vi "SubVI Nivel a Caudal peristaltica.vi"(11 "UInt16":u16) -> (3 "Numeric":dbl)   [LabVIEW 2013]
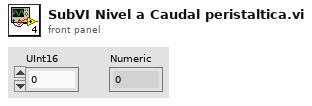
[diagram p1: front panel]
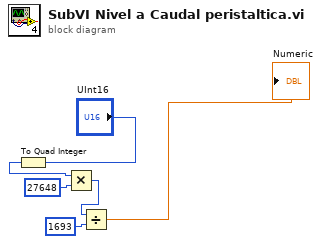
[diagram p0: block diagram]
diagram:
  n1 = To Quad Integer(1:"UInt16") -> ()  [unwired: 1 out]
  n2 = Multiply(x="UInt16", y=27648) -> (x*y=w4:i32)
  n3 = Divide(x=w4, y=1693) -> (x/y=→"Numeric":dbl)
